vi "Conn Set Properties.vi"(4 "error in (no error)":errorcluster, 5 "connection properties":T1, 7 "connection reference":T2) -> (0 "error out":errorcluster, 3 "connection reference out":T2)   [LabVIEW 2017, in "NI_Database_API.lvlib"]
doc: "Sets properties on the object as determined by the inputs. Wire data to the reference and properties inputs to determine the polymorphic instance to use or manually select the instance."
uses:
  <vilib>/addons/database/NI_Database_API.lvlib
  <vilib>/addons/database/Connection.llb/Conn ObjectReference.ctl
  <vilib>/addons/database/Connection.llb/Conn Properties.ctl
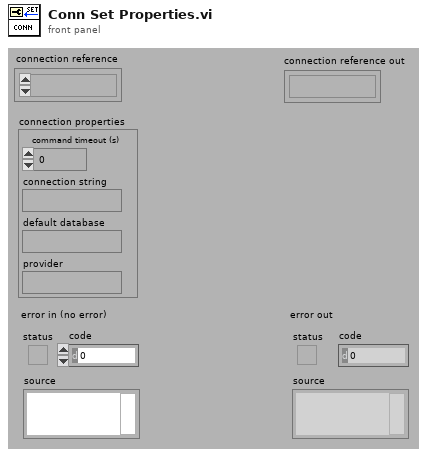
[diagram p1: front panel]
types:
  T1 = typedef "NI_Database_API.lvlib/Conn Properties.ctl" = cluster{"command timeout (s)":i32, "connection string":string, "default database":string, "provider":string}
  T2 = typedef "NI_Database_API.lvlib/Conn ObjectReference.ctl" = refnum<k1>
  T3 = typedef "NI_Database_API.lvlib/Conn DataMembers.ctl" = cluster{"ADODB._Connection":refnum<k7>, "recordset objects":i32, "command objects":i32}
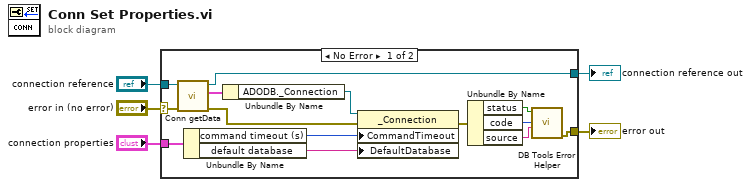
[diagram p0: block diagram]
diagram:
  n1 = case shown="No Error" "error in (no error)" {
    selector: "error in (no error)" -> [w6 w21]
    tunnel: "connection properties" -> [w18 _]
    tunnel: "connection reference" -> [w14 w20]
    tunnel: [w13 w20] -> w3
    tunnel: [w7 w21] -> w2
    frame No Error {
      n2 = call <vilib>:"Conn getData.vi"("error in (no error)"=w6, "connection reference"=w14) -> ("error out"=w12:errorcluster, "data"=w15:T3, "connection reference out"=w13:T2)  [unwired: 3 out]
      n3 = Unbundle By Name(w18) -> ("command timeout (s)"=w17:i32, "default database"=w16:string)
      n4 = Unbundle By Name(w15) -> ("ADODB._Connection"=w19:refnum<k7>)
      n5 = property class="_Connection"(reference=w19, error in=w12, "CommandTimeout"=w17, "DefaultDatabase"=w16) -> (error out=w8:errorcluster)  [unwired: 1 out]
      n6 = Unbundle By Name(w8) -> ("status"=w10:bool, "code"=w9:i32, "source"=w11:string)
      n7 = call <vilib>:"DB Tools Error Helper.vi"("source"=w11, "code"=w9, "status"=w10) -> ("error out"=w7:errorcluster)  [unwired: 1 in, 7 out]
    }
    frame Error {
    }
  }
  "connection reference out" <- w3
  "error out" <- w2
